vi "Demo_CLOSE_SQL_DATA.vi"(8 "error in (no error)":errorcluster, 9 "TABLE NAME":string, 10 "CONDITION string":string, 11 "Refnum in":T1) -> (0 "error out":errorcluster, 3 "Refnum out":T1)   [LabVIEW 2017]
uses:
  <vilib>/addons/database/Connection.llb/Conn ObjectReference.ctl
  <vilib>/addons/database/NI_Database_API.lvlib
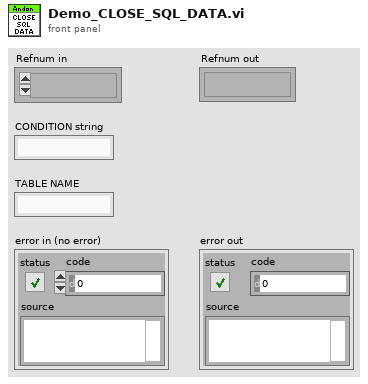
[diagram p1: front panel]
types:
  T1 = typedef "NI_Database_API.lvlib/Conn ObjectReference.ctl" = refnum<k1>
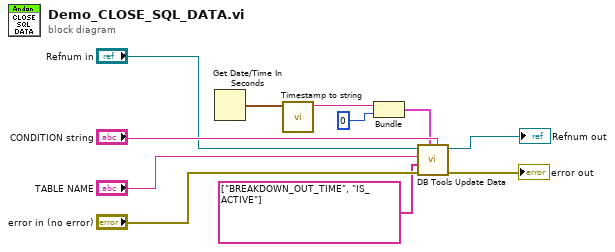
[diagram p0: block diagram]
diagram:
  n1 = Get Date/Time In Seconds() -> (seconds since 1Jan1904=w9:timestamp)
  n2 = call "Timestamp to string.vi"("time stamp"=w9) -> ("date/time string"=w1:string)  [unwired: 8 in, 2 out]
  n3 = Bundle("date/time string"=w1, 0) -> (w3:cluster{"date/time string":string, i32})  [unwired: 1 in]
  n4 = call <vilib>:"DB Tools Update Data.vi"("condition"="CONDITION string", "data"=w3, "error in (no error)"="error in (no error)", "columns"=string[] ["BREAKDOWN_OUT_TIME", "IS_ACTIVE"], "table"="TABLE NAME", "connection reference"="Refnum in") -> ("error out"=→"error out":errorcluster, "connection reference out"=→"Refnum out":T1)  [unwired: 4 in]
